vi "Read.vi"(4 "error in (no error)":errorcluster, 7 "Device handle in":u32 format="%x") -> (0 "error out":errorcluster, 1 "Rel. humidity (%)":dbl, 2 "Temperature (°C)":dbl, 3 "Device handle out":u32 format="%x")   [LabVIEW 2014, in "MBUG-2820.lvlib"]
doc: "Performs a single, new measurement of temperature an relativehumidity."
uses:
  <instrlib>/MBUG-2820/MBUG-2820.lvlib
  <instrlib>/MBUG-2820/mbugdll.dll
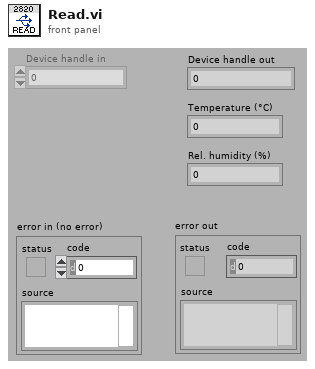
[diagram p1: front panel]
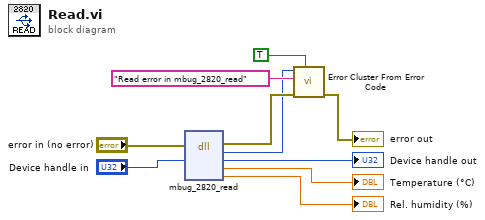
[diagram p0: block diagram]
diagram:
  n1 = dll-call lib="C:/Programme/National Instruments/LabVIEW 2014/instr.lib/MBUG-2820/mbugdll.dll" fn="mbug_2820_read"(error in="error in (no error)", "dev_handle"="Device handle in") -> (error out=w5:errorcluster, "return"=w1:i32, "dev_handle"=→"Device handle out":u64, "temperature"=→"Temperature (°C)":dbl, "humidity"=→"Rel. humidity (%)":dbl)  [unwired: 4 in, 1 out]
  n2 = call <vilib>:"Error Cluster From Error Code.vi"("show call chain? (False)"=TRUE, "error in (no error)"=w5, "error message (\"\")"="Read error in mbug_2820_read", "error code (0)"=w1) -> ("error out"=→"error out":errorcluster)  [unwired: 5 in]
